vi "createAVIRefnum.vi"(8 "error in":errorcluster, 10 "Video filename":string, 11 "Input cluster":T1) -> (0 "error out":errorcluster, 3 "Output cluster":T1)   [LabVIEW 2020]
uses:
  controls/StateMachineVariables.ctl
  <vilib>/vision/Avi.llb/IMAQ AVI2 Refnum.ctl
  <vilib>/userDefined/High Color/IMAQdx.ctl
  <vilib>/vision/Deep Learning.llb/IMAQ DL Model Refnum.ctl
  <vilib>/vision/Image Controls.llb/IMAQ Image.ctl
  <vilib>/vision/Avi.llb/IMAQ AVI2 Codec Path.ctl
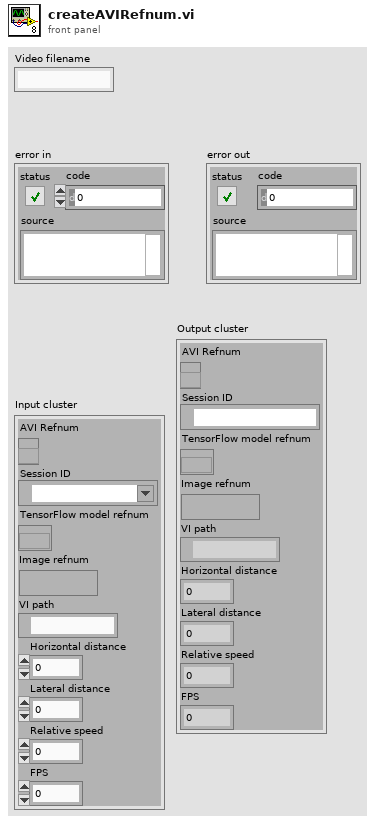
[diagram p1: front panel]
types:
  T1 = typedef "StateMachineVariables.ctl" = cluster{"AVI Refnum":T2, "Session ID":T3, "TensorFlow model refnum":T4, "Image refnum":T5, "VI path":path, "Horizontal distance":dbl, "Lateral distance":dbl, "Relative speed":dbl, "FPS":dbl}
  T2 = typedef "IMAQ AVI2 Refnum.ctl" = refnum<k20>
  T3 = typedef "IMAQdx.ctl" = refnum<k21>
  T4 = typedef "IMAQ DL Model Refnum.ctl" = refnum<k20>
  T5 = typedef "IMAQ Image.ctl" = refnum<image>
  T6 = typedef "IMAQ AVI2 Codec Path.ctl" = u32
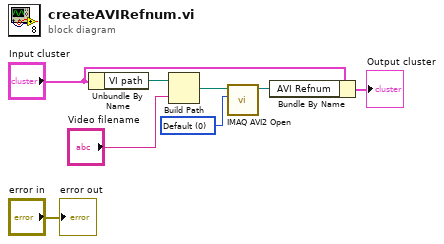
[diagram p0: block diagram]
diagram:
  w6 = T6 0 items=["Default", "System", "Built in Vision"] ("Codec Source")
  n1 = Unbundle By Name("Input cluster") -> ("VI path"=w1:path)
  n2 = Build Path(base path=w1, name or relative path="Video filename") -> (appended path=w7:path)
  n3 = call "IMAQ AVI2 Open"("Codec Source"=w6, "AVI File Path"=w7) -> ("AVI Refnum"=w3:T2)  [unwired: 8 in, 1 out]
  n4 = Bundle By Name(cluster="Input cluster", "AVI Refnum"=w3) -> (→"Output cluster":T1)
  "error out" <- "error in"
